vi "Joystick - Begin All.vi"(4 "Right Joystick Port":T1=enum."USB 1", 5 "Left Joystick Name":string="Left Joystick", 6 "Right Joystick Name":string="Right Joystick", 7 "Left Joystick Port":T1, 8 "error in (no error)":errorcluster) -> (0 "error out":errorcluster)   [LabVIEW 2015]
uses:
  <vilib>/Rock Robotics/WPI/Joystick/WPI_JoystickDeviceEnum.ctl
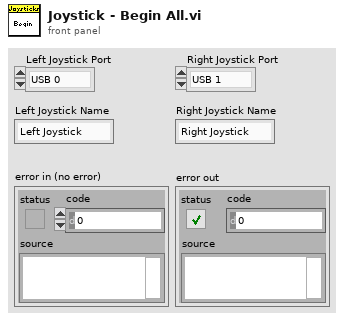
[diagram p1: front panel]
types:
  T1 = typedef "WPI_JoystickDeviceEnum.ctl" = enum16{"USB 0", "USB 1", "USB 2", "USB 3", "USB 4", "USB 5"}
  T2 = typedef "WPI_JoystickDevRef.ctl" = cluster{"Device":T1}
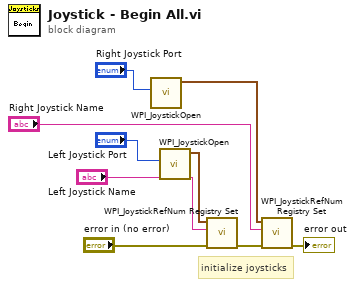
[diagram p0: block diagram]
diagram:
  # "initialize joysticks"
  n1 = call <vilib>:"WPI_JoystickOpen.vi"("JoystickDevice"="Right Joystick Port") -> ("JoystickDevRef"=w6:T2)  [unwired: 10 in]
  n2 = call <vilib>:"WPI_JoystickOpen.vi"("JoystickDevice"="Left Joystick Port") -> ("JoystickDevRef"=w3:T2)  [unwired: 10 in]
  n3 = call <vilib>:"WPI_JoystickRefNum Registry Set.vi"("error in (no error)"="error in (no error)", "refnum name"="Left Joystick Name", "JoystickDevRef"=w3) -> ("error out"=w8:errorcluster)  [unwired: 7 in, 1 out]
  n4 = call <vilib>:"WPI_JoystickRefNum Registry Set.vi"("error in (no error)"=w8, "refnum name"="Right Joystick Name", "JoystickDevRef"=w6) -> ("error out"=→"error out":errorcluster)  [unwired: 7 in, 1 out]
